vi "WritePathloss.vi"() -> ()   [LabVIEW 2015]
uses:
  PhyPort.ctl
  VISAOperation.ctl
panel:
  in  "PathlossConfig":T2={"PathlossFilePath"=path "D:/4-Up-WLAN-Test-System/WTSInstrumentControl/Pathloss/External Pathloss.txt", "Pathloss Table Name"="wlan", "PhyPort"=enum."Port5"}
  in  "VISA resource name":refnum<visa-resource-name>="TCPIP0::10.144.41.54::inst0::INSTR"
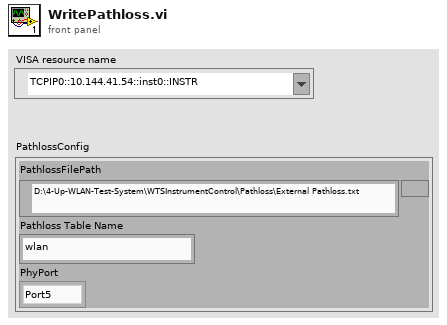
[diagram p1: front panel]
types:
  T1 = typedef "PhyPort.ctl" = enum16{"Port0", "Port1", "Port2", "Port3", "Port4", "Port5", "Port6", "Port7"}
  T2 = cluster{"PathlossFilePath":path, "Pathloss Table Name":string, "PhyPort":T1}
  T3 = typedef "VISAOperation.ctl" = enum16{"RunFile", "OpenDebugPanel", "ReadError", "ReadSTB", "Reset", "Clean", "CloseVISA", "RunCMD", "OpenVISA"}
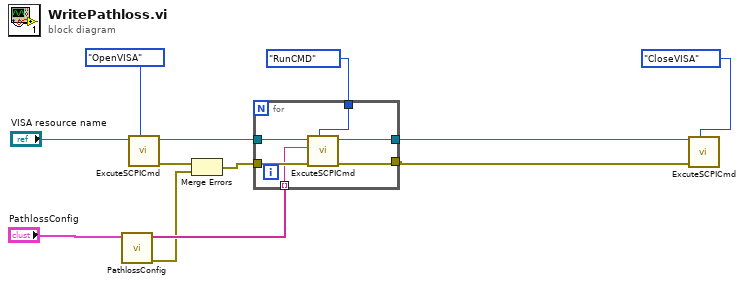
[diagram p0: block diagram]
diagram:
  n1 = call "PathlossConfig.vi"("PathlossConfig"="PathlossConfig") -> ("error out"=w1:errorcluster, "PahtlossCMD"=w4:string[])  [unwired: 9 in]
  n2 = call "ExcuteSCPICmd.vi"("VISAOperation"=VISAOperation."OpenVISA", "VISA resource name"="VISA resource name") -> ("error out"=w9:errorcluster, "reference out"=w8:refnum<visa-resource-name>)  [unwired: 6 in, 2 out]
  n3 = Merge Errors(w9, w1) -> (w6:errorcluster)
  n4 = for {
    tunnel: VISAOperation."RunCMD" ("VISAOperation") -> [w16]
    tunnel: w8 -> [w18]
    tunnel: [w17] -> w3
    tunnel: w6 -> [w15]
    tunnel: [w14] -> w2
    tunnel: w4 -> [w13] mode=indexing
    n5 = call "ExcuteSCPICmd.vi"("VISAOperation"=w16, "error in (no error)"=w15, "Run Command"=w13, "VISA resource name"=w18) -> ("error out"=w14:errorcluster, "reference out"=w17:refnum<visa-resource-name>)  [unwired: 4 in, 2 out]
  }
  n6 = call "ExcuteSCPICmd.vi"("VISAOperation"=VISAOperation."CloseVISA", "error in (no error)"=w2, "VISA resource name"=w3) -> ()  [unwired: 5 in, 4 out]
